vi "Filter_String_Parser.vi"(11 "Filter String":string="Protocol == UDP AND Length > 0.7 OR Source == 192.168.1.1") -> (1 "Comparators":T1(array[cluster]), 3 "Boolean Connectors":string[](array[string]))   [LabVIEW 2025]
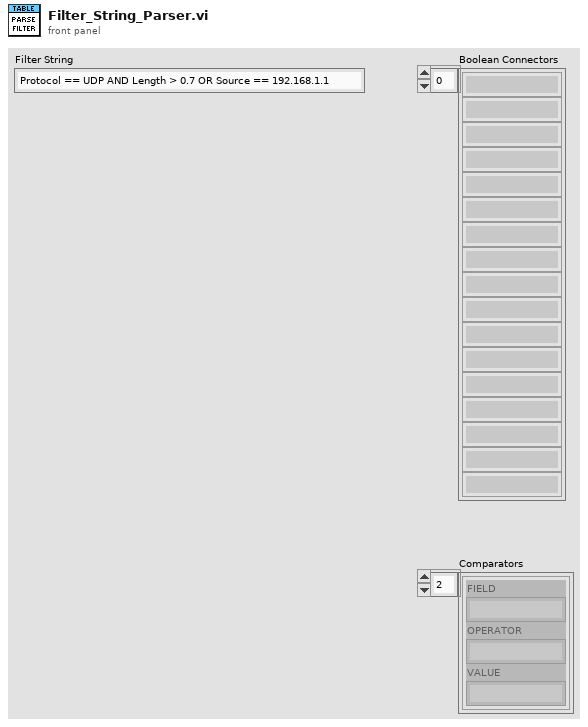
[diagram p1: front panel]
types:
  T1 = cluster{"FIELD":string, "OPERATOR":string, "VALUE":string}[]
  T2 = cluster{"FIELD":string, "OPERATOR":string, "VALUE":string}
  T3 = enum16{"Packet Number", "Timestamp", "Source", "Destination", "Protocol", "Length", "Data"}
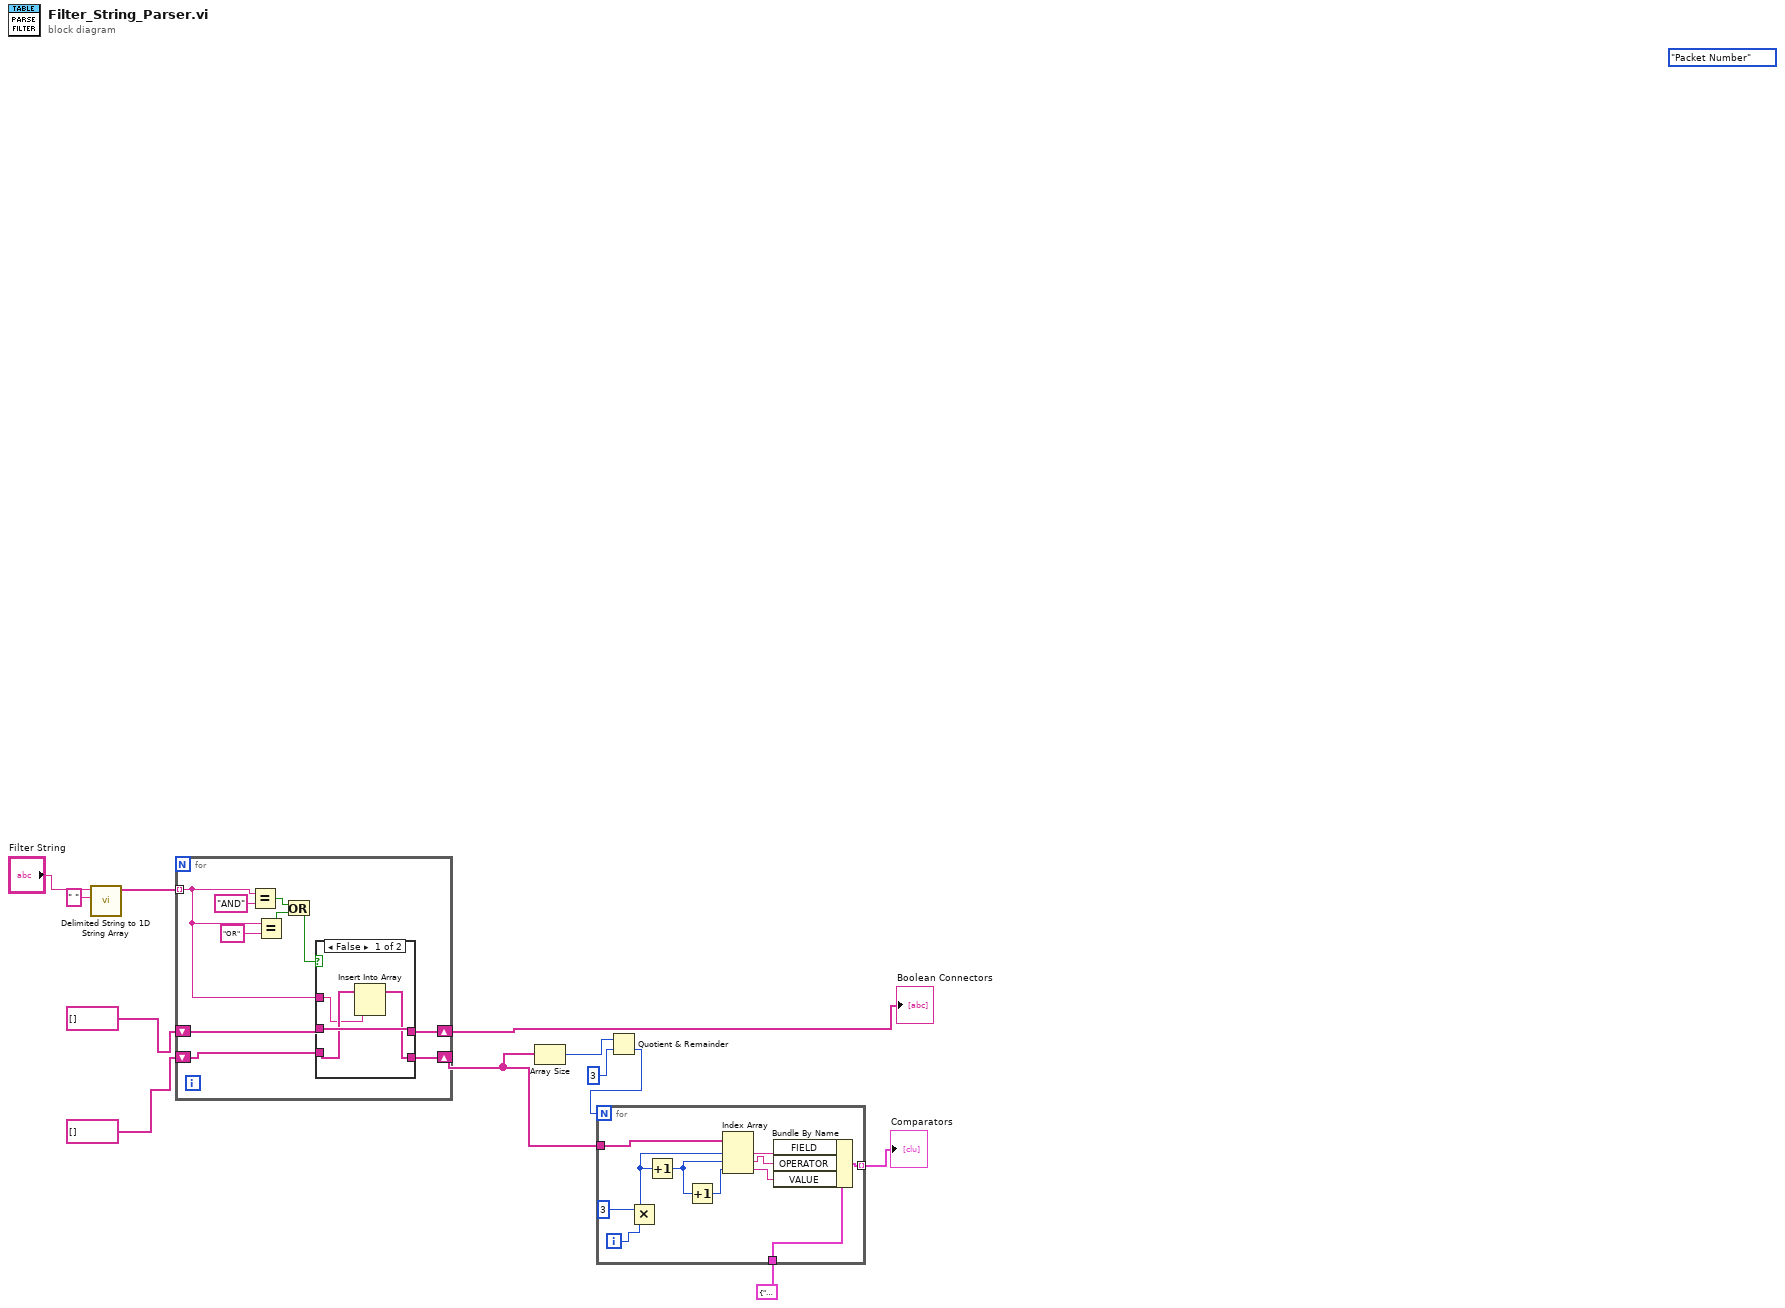
[diagram p0: block diagram]
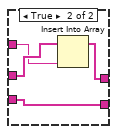
[diagram p2: hidden frame]
diagram:
  (unwired) T3."Packet Number" ("Sort By")
  n1 = call <vilib>:"Delimited String to 1D String Array.vi"("delimiter"=" ", "delimited string"="Filter String") -> ("string array"=w10:string[])  [unwired: 9 in]
  n2 = for {
    tunnel: w10 -> [w17] mode=indexing
    shift-right: [w13] -> w4
    shift-left: string[] [] -> [w16]
    shift-right: [w14] -> w3
    shift-left: string[] [] -> [w15]
    n3 = Equal?(x=w17, y="AND") -> (x = y?=w22:bool)
    n4 = Equal?(x=w17, y="OR") -> (x = y?=w19:bool)
    n5 = Or(x=w22, y=w19) -> (x .or. y?=w18:bool)
    n6 = case shown="False" w18 {
      tunnel: w17 -> [w24 w28]
      tunnel: w16 -> [w26 w29]
      tunnel: [w26 w27] -> w13
      tunnel: w15 -> [w25 w30]
      tunnel: [w23 w30] -> w14
      frame False {
        n7 = Insert Into Array(array=w25, new element=w24) -> (w23:string[])  [unwired: 1 in]
      }
      frame True {
        n8 = Insert Into Array(array=w29, new element=w28) -> (w27:string[])  [unwired: 1 in]
      }
    }
  }
  "Boolean Connectors" <- w4
  n9 = Array Size(array=w3) -> (size(s)=w8:i32)
  n10 = Quotient & Remainder(x=w8, y=3) -> (floor(x/y)=w1:i32)  [unwired: 1 out]
  n11 = for {
    N: w1 -> [_]
    tunnel: w3 -> [w41]
    tunnel: T2 {"FIELD"="", "OPERATOR"="", "VALUE"=""} -> [w35]
    tunnel: [w31] -> w6 mode=indexing
    i -> [w40]
    n12 = Multiply(x=3, y=w40) -> (x*y=w38:i32)
    n13 = Increment(x=w38) -> (x+1=w36:i32)
    n14 = Increment(x=w36) -> (x+1=w37:i32)
    n15 = Index Array(array=w41, index #1=w38, index #2=w36, index #3=w37) -> (element #1=w34:string, element #2=w33:string, element #3=w32:string)
    n16 = Bundle By Name(cluster=w35, "FIELD"=w34, "OPERATOR"=w33, "VALUE"=w32) -> (w31:T2)
  }
  "Comparators" <- w6
